vi "incrementar_CheckfinalQR.vi"(8 "error in (no error)":errorcluster, 11 "TEST ASICS INPUT":T1) -> (0 "error out":errorcluster, 1 "output cluster":T1={"COORD X"=0, "COORD  Y"=0, "NºASICS"=1, "SELECCIÓN DE BANDEJA"=enum."BANDEJA ENTRADA", "CONTEO QR"=0}, 2 "FINAL ASICS??":bool, 3 "Asics pendientes":u32)   [LabVIEW 2019]
uses:
  TYPE'S DEF/INPUT LECTURA_QR.ctl
panel:
  # "CELDA DE COMIENZO"
  # "CELDA DE COMIENZO"
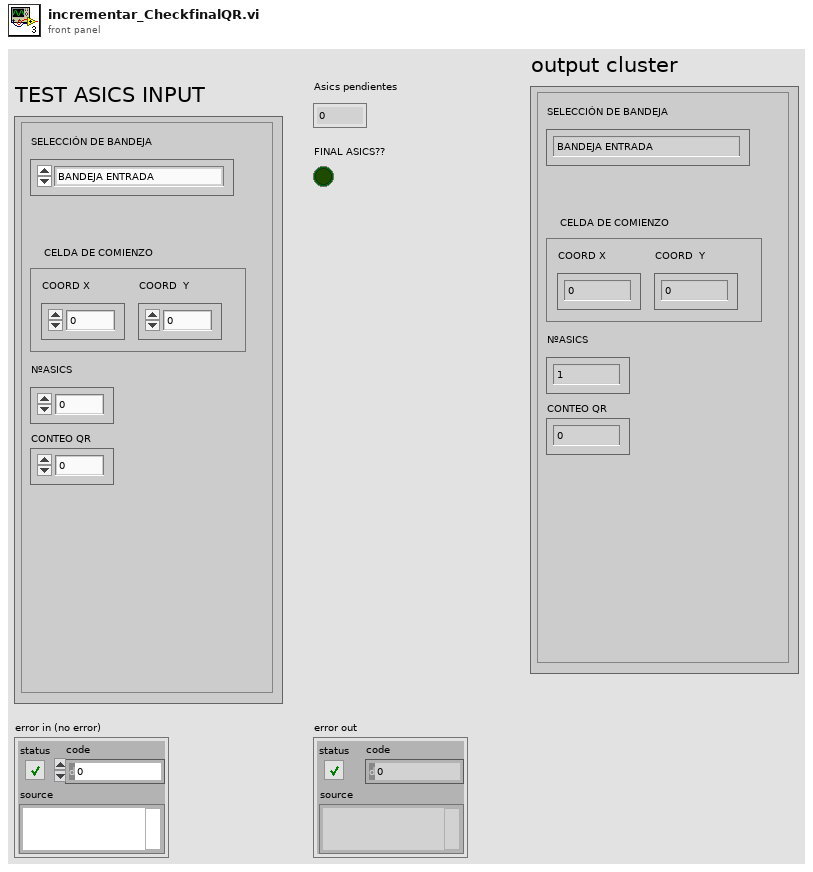
[diagram p1: front panel]
types:
  T1 = typedef "INPUT LECTURA_QR.ctl" = cluster{"COORD X":u16, "COORD  Y":u16, "NºASICS":u32, "SELECCIÓN DE BANDEJA":enum16{"BANDEJA ENTRADA", "BANDEJA OK", "BANDEJA NOK"}, "CONTEO QR":u32}
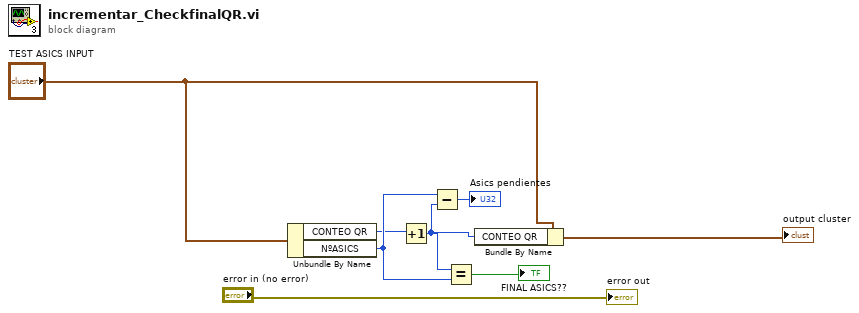
[diagram p0: block diagram]
diagram:
  n1 = Unbundle By Name("TEST ASICS INPUT") -> ("CONTEO QR"=w5:u32, "NºASICS"=w8:u32)
  n2 = Increment(x=w5) -> (x+1=w7:u32)
  n3 = Subtract(x=w8, y=w7) -> (x-y=→"Asics pendientes":u32)
  n4 = Equal?(x=w7, y=w8) -> (x = y?=→"FINAL ASICS??":bool)
  n5 = Bundle By Name(cluster="TEST ASICS INPUT", "CONTEO QR"=w7) -> (→"output cluster":T1)
  "error out" <- "error in (no error)"
